vi "PC_TDMS_reader.vi"() -> ()   [LabVIEW 2020]
panel:
  out "XY Graph":cluster{"Ramp Pattern":dbl[], "magnitude":dbl[]}(graph)
  out "Waveform Graph":waveform(dbl)(graph)
  in  "Boolean":bool
  in  "Path":path
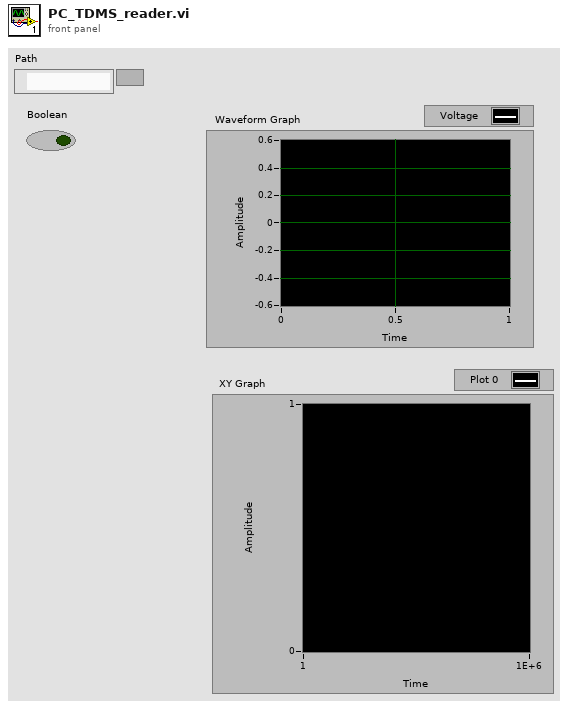
[diagram p1: front panel]
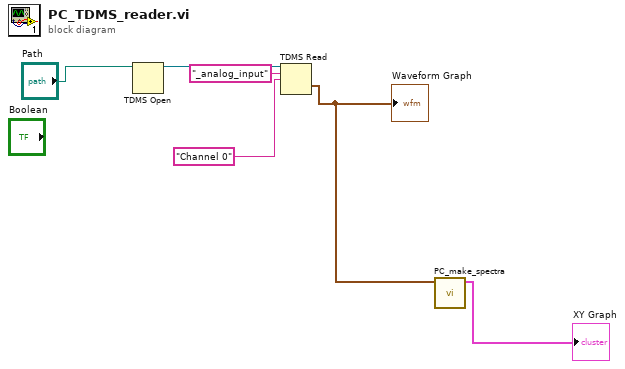
[diagram p0: block diagram]
diagram:
  n1 = TDMS Open(11:"Path") -> (3:w5:refnum<k34>)  [unwired: 6 in, 1 out]
  n2 = TDMS Read(0:w5, 5:"_analog_input" ("group name in"), 7:"Channel 0" ("group name in")) -> (10:w2:waveform(dbl))  [unwired: 5 in, 5 out]
  "Waveform Graph" <- w2
  n3 = call "PC_make_spectra.vi"("waveform in"=w2) -> ("Cluster"=→"XY Graph":cluster{"Ramp Pattern":dbl[], "magnitude":dbl[]})  [unwired: 9 in, 1 out]
